vi "BLE_Read_CharacteristicArray.vi"(0 ".NET Refnum in":refnum<k24>, 5 "ServicesUUIDs Extract Value":string[](array[string]), 11 "error in (no error)":errorcluster) -> (4 ".NET Refnum out":refnum<k24>, 6 "ServicesUUIDs ASCII Value":string[](array[string]), 8 "ServicesUUIDs Value":string[](array[string]), 15 "error out":errorcluster)   [LabVIEW 2020, in "BLE.lvlib"]
uses:
  C:/Users/Trait/Desktop/LabView Project/LabView BLE DataACQ/BLELib.dll
  BLELib.dll
  BLE.lvlib
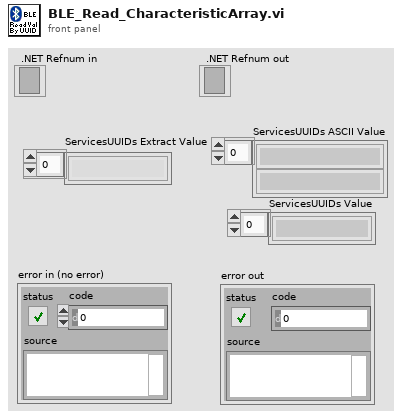
[diagram p1: front panel]
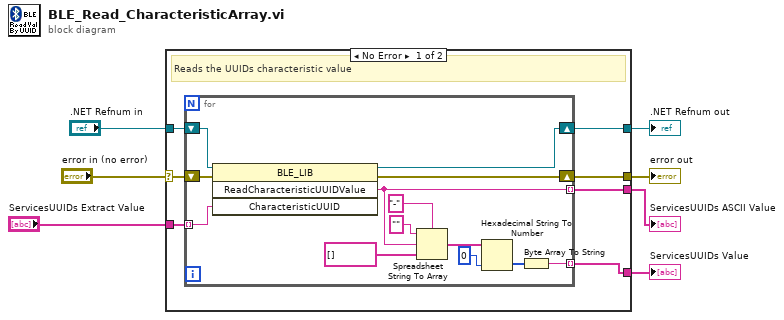
[diagram p0: block diagram]
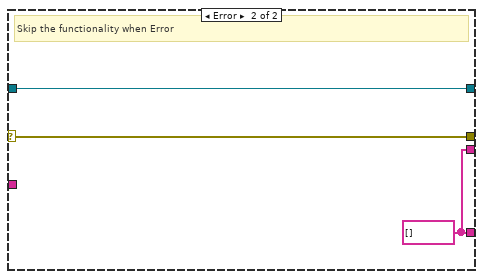
[diagram p2: hidden frame]
diagram:
  n1 = case shown="No Error" "error in (no error)" {
    selector: "error in (no error)" -> [w14 w29]
    tunnel: [w13 w30] -> w6
    tunnel: ".NET Refnum in" -> [w12 w30]
    tunnel: [w11 w29] -> w4
    tunnel: "ServicesUUIDs Extract Value" -> [w10 _]
    tunnel: [w9 w28] -> w2
    tunnel: [w8 w28] -> w1
    frame No Error {
      # "Reads the UUIDs characteristic value"
      n2 = for {
        shift-right: [w16] -> w11
        shift-left: w14 -> [w27]
        shift-right: [w26] -> w13
        shift-left: w12 -> [w25]
        tunnel: w10 -> [w17] mode=indexing
        tunnel: [w15] -> w9 mode=indexing
        tunnel: [w18] -> w8 mode=indexing
        n3 = invoke class="BLE_LIB" method="ReadCharacteristicUUIDValue"(reference=w25, error in=w27, "CharacteristicUUID"=w17) -> (reference out=w26:refnum<k24>, error out=w16:errorcluster, "ReadCharacteristicUUIDValue"=w15:string)  [unwired: 1 in, 1 out]
        n4 = Spreadsheet String To Array(delimiter (Tab)="-", format string="", spreadsheet string=w15, array type (2D Dbl)=string[] []) -> (array=w21:string[])
        n5 = Hexadecimal String To Number(string=w21, default (0uL)=u8 0 ("default (0 U32)")) -> (number=w19:u8[])  [unwired: 1 in, 1 out]
        n6 = Byte Array To String(unsigned byte array=w19) -> (string=w18:string)
      }
    }
    frame Error {
      w28 = string[] []
      # "Skip the functionality when Error"
    }
  }
  "error out" <- w4
  ".NET Refnum out" <- w6
  "ServicesUUIDs ASCII Value" <- w2
  "ServicesUUIDs Value" <- w1
